vi "Empty Data Check.vi"(11 "Cluster Data":T4) -> (3 "Empty?":bool)   [LabVIEW 2021]
uses:
  IP Simulation/Controls/IP_Cellular Tech Type def.ctl
  IP Simulation/Controls/IP_Network_Type def.ctl
  IP Simulation/Controls/IP_Type-Tydedef.ctl
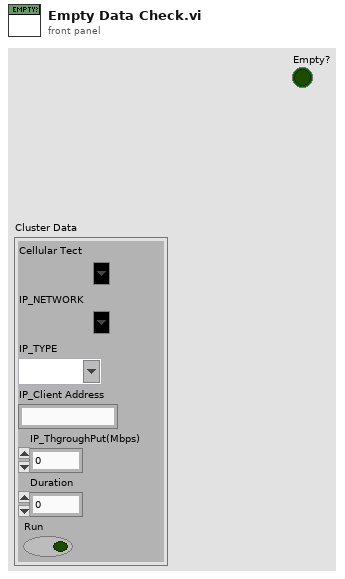
[diagram p1: front panel]
types:
  T1 = typedef "IP_Cellular Tech Type def.ctl" = string
  T2 = typedef "IP_Network_Type def.ctl" = string
  T3 = typedef "IP_Type-Tydedef.ctl" = string
  T4 = cluster{"Cellular Tect":T1, "IP_NETWORK":T2, "IP_TYPE":T3, "IP_Client Address":string, "IP_ThgroughPut(Mbps)":i32, "Duration":i32, "Run":bool}
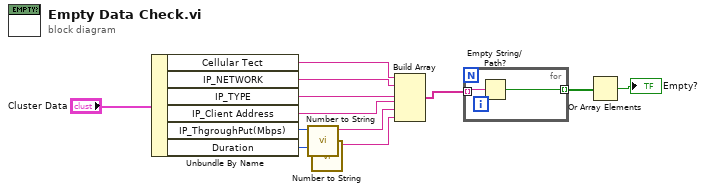
[diagram p0: block diagram]
diagram:
  n1 = Unbundle By Name("Cluster Data") -> ("Cellular Tect"=w4:T1, "IP_NETWORK"=w5:T2, "IP_TYPE"=w6:T3, "IP_Client Address"=w7:string, "IP_ThgroughPut(Mbps)"=w11:i32, "Duration"=w10:i32)
  n2 = call "Number to String.vi"("DecimaL NU\nmber"=w11) -> ("Decimal String"=w8:string)  [unwired: 10 in]
  n3 = call "Number to String.vi"("DecimaL NU\nmber"=w10) -> ("Decimal String"=w9:string)  [unwired: 10 in]
  n4 = Build Array(w4, w5, w6, w7, w8, w9) -> (w3:T3[])
  n5 = for {
    tunnel: w3 -> [w14] mode=indexing
    tunnel: [w13] -> w2 mode=indexing
    n6 = Empty String/Path?(string/path=w14) -> (empty?=w13:bool)
  }
  n7 = Or Array Elements(Boolean array=w2) -> (logical OR=→"Empty?":bool)
